vi "Vibration.vi"() -> ()   [LabVIEW 2012]
uses:
  <vilib>/measure/madcrms.llb/Basic Averaged DC-RMS for 1 Chan.vi
  <vilib>/measure/NI_MAPro.lvlib
panel:
  out "选项卡":T1(tab)
  in  "装置IP":string
  in  "?":bool
  in  "灵敏度(mv/g)":u16=1 min=1
  in  "采样率(ksps)":T2(ring)
  in  "?":bool
  in  "?":bool
  in  "开始":bool
  in  "?":bool
  in  "设置装置网关":string
  in  "设置装置子网掩码":string
  in  "设置装置IP":string
  in  "?":bool
  in  "是否开启电流源":u8(knob) scale=0.0..1.0
  in  "是否进行自校准":u8(knob) scale=0.0..1.0
  in  "?":bool
  in  "?":path
  in  "是否保存数据":u8(knob) scale=0.0..1.0
  in  "?":bool
  out "进度条":dbl(slide) scale=0.0..99.0
  out "字符串":string
  out "波形卡":enum32{"波形卡 1", "波形卡 2", "波形卡 3"}(tab)
  in  "AC/DC":bool
  in  "Y轴调整":dbl(knob)=1.0 min=0.0001 max=5.5 step=0.001 scale=0.0001..5.5
  out "?":dbl[](graph)
  out "?":dbl[](graph)
  in  "X轴调整":u16(knob)=50 min=50 max=50000 scale=50.0..50000.0
  in  "列表框":i32(listbox)
  out "?":u16[](graph)
  out "转 \n速":u16(knob) scale=0.0..20000.0
  # "PageUp\nPageDown\n微调"
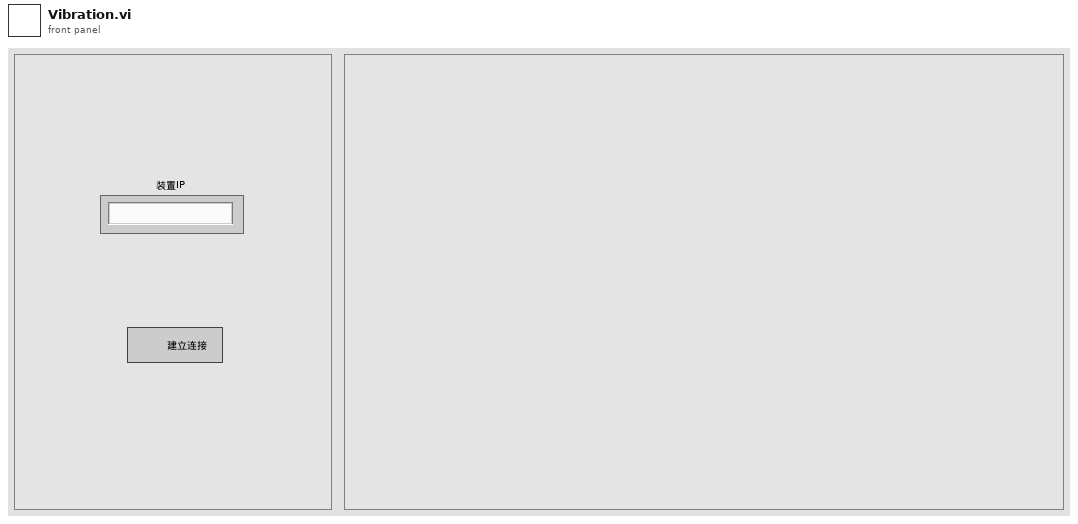
[diagram p1: front panel]
types:
  T1 = enum32{"选项卡 1", "选项卡 2", "选项卡 3", "选项卡 4", "选项卡 5", "选项卡 6", "选项卡 7"}
  T2 = enum16{"105.468", "52.734", "35.156", "26.367", "21.094", "17.578", "15.067", "13.184", "11.719", "10.545"}
  T3 = enum8{"Enabled", "Disabled", "Disabled and Grayed Out"}
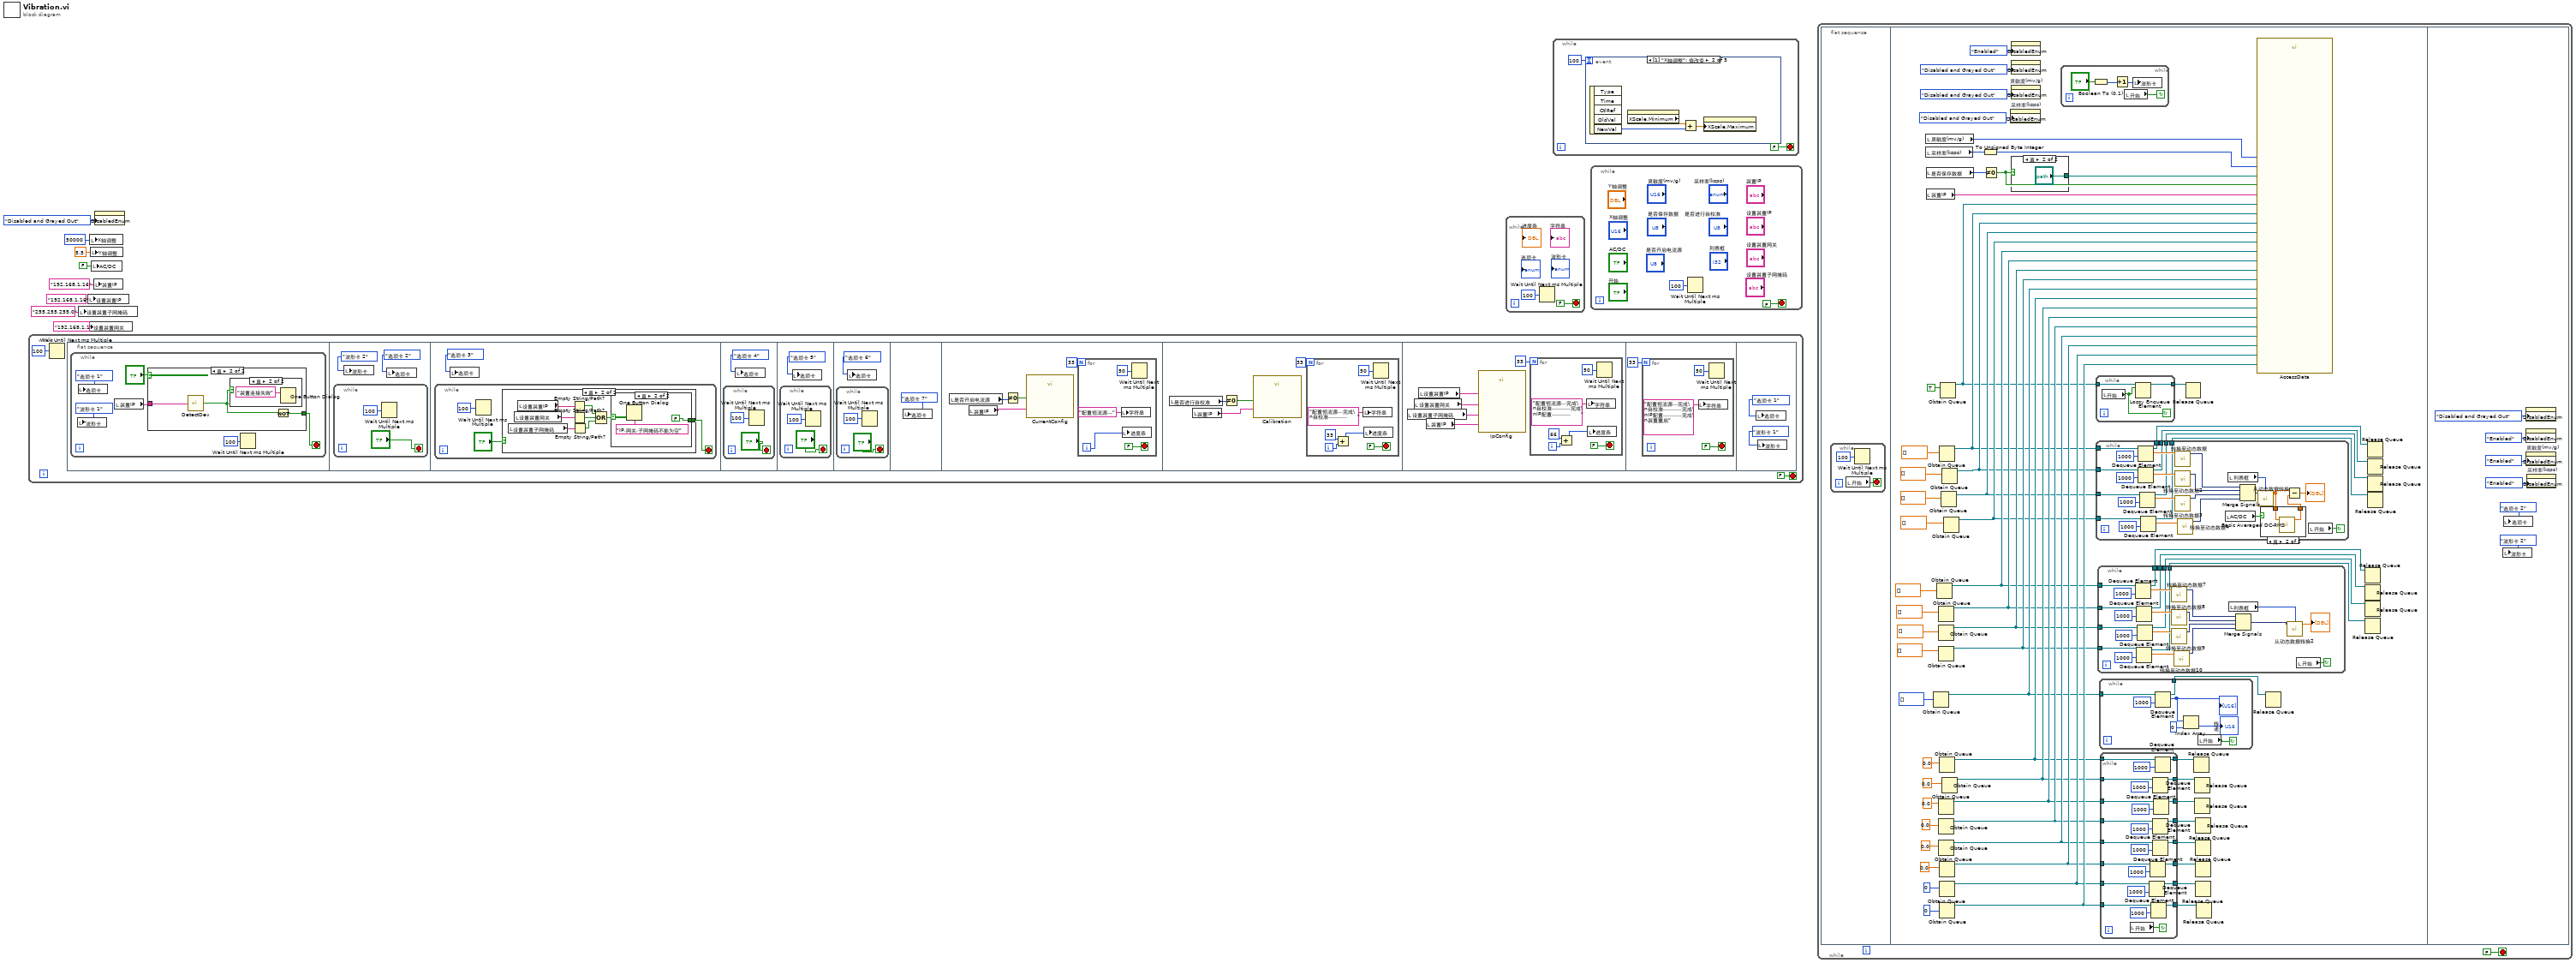
[diagram p0: block diagram]
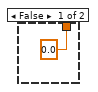
[diagram p2: hidden frame]
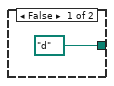
[diagram p3: hidden frame]
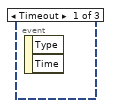
[diagram p4: hidden frame]
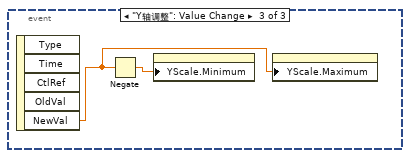
[diagram p5: hidden frame]
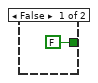
[diagram p6: hidden frame]
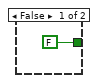
[diagram p8: hidden frame]
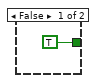
[diagram p9: hidden frame]
diagram:
  n1 = while {
    stop <- FALSE stop-if-true
    n2 = Wait Until Next ms Multiple(millisecond multiple=u32 100 ("毫秒倍数")) -> ()  [unwired: 1 out]
    n3 = flat-sequence {
      frame #0 {
        n4 = while {
          stop <- w15 stop-if-true
          n5 = local write "波形卡"(enum32{"波形卡 1", "波形卡 2", "波形卡 3"}."波形卡 1" ("波形卡")) -> ()
          n6 = local write "选项卡"(T1."选项卡 1" ("选项卡")) -> ()
          n7 = local read "装置IP"() -> (w11:string)
          n8 = case shown="真" "?" {
            tunnel: [FALSE w20] -> w15
            tunnel: w11 -> [_ w18]
            frame False {
            }
            frame True {
              n9 = call "DetectDev.vi"("IP."=w18) -> ("Fail"=w19:bool)
              n10 = case shown="真" w19 {
                frame False {
                }
                frame True {
                  n11 = One Button Dialog(message="装置连接失败" ("消息")) -> ()  [unwired: 1 in, 1 out]
                }
              }
              n12 = Not(x=w19) -> (.not. x?=w20:bool)
            }
          }
          n13 = Wait Until Next ms Multiple(millisecond multiple=u32 100 ("毫秒倍数")) -> ()  [unwired: 1 out]
        }
      }
      frame #1 {
        n14 = while {
          stop <- "?" stop-if-true
          n15 = Wait Until Next ms Multiple(millisecond multiple=u32 100 ("毫秒倍数")) -> ()  [unwired: 1 out]
        }
        n16 = local write "波形卡"(enum32{"波形卡 1", "波形卡 2", "波形卡 3"}."波形卡 2" ("波形卡")) -> ()
        n17 = local write "选项卡"(T1."选项卡 2" ("选项卡")) -> ()
      }
      frame #2 {
        n18 = while {
          stop <- w27 stop-if-true
          n19 = Wait Until Next ms Multiple(millisecond multiple=u32 100 ("毫秒倍数")) -> ()  [unwired: 1 out]
          n20 = case shown="真" "?" {
            tunnel: [FALSE w31] -> w27
            frame False {
            }
            frame True {
              n21 = local read "设置装置子网掩码"() -> (w38:string)
              n22 = local read "设置装置网关"() -> (w37:string)
              n23 = local read "设置装置IP"() -> (w36:string)
              n24 = Empty String/Path?(string/path=w36) -> (empty?=w33:bool)
              n25 = Empty String/Path?(string/path=w37) -> (empty?=w34:bool)
              n26 = Empty String/Path?(string/path=w38) -> (empty?=w35:bool)
              n27 = Compound Arithmetic op=OR(w33, w34, w35) -> (w32:bool)
              n28 = case shown="真" w32 {
                tunnel: [TRUE FALSE] -> w31
                frame False {
                }
                frame True {
                  n29 = One Button Dialog(message="IP,网关,子网掩码不能为空" ("消息")) -> ()  [unwired: 1 in, 1 out]
                }
              }
            }
          }
        }
        n30 = local write "选项卡"(T1."选项卡 3" ("选项卡")) -> ()
      }
      frame #3 {
        n31 = while {
          stop <- "?" stop-if-true
          n32 = Wait Until Next ms Multiple(millisecond multiple=u32 100 ("毫秒倍数")) -> ()  [unwired: 1 out]
        }
        n33 = local write "选项卡"(T1."选项卡 4" ("选项卡")) -> ()
      }
      frame #4 {
        n34 = while {
          stop <- "?" stop-if-true
          n35 = Wait Until Next ms Multiple(millisecond multiple=u32 100 ("毫秒倍数")) -> ()  [unwired: 1 out]
        }
        n36 = local write "选项卡"(T1."选项卡 5" ("选项卡")) -> ()
      }
      frame #5 {
        n37 = while {
          stop <- "?" stop-if-true
          n38 = Wait Until Next ms Multiple(millisecond multiple=u32 100 ("毫秒倍数")) -> ()  [unwired: 1 out]
        }
        n39 = local write "选项卡"(T1."选项卡 6" ("选项卡")) -> ()
      }
      frame #6 {
        n40 = local write "选项卡"(T1."选项卡 7" ("选项卡")) -> ()
      }
      frame #7 {
        n41 = local read "是否开启电流源"() -> (w53:u8)
        n42 = local read "装置IP"() -> (w52:string)
        n43 = Not Equal To 0?(x=w53) -> (x != 0?=w54:bool)
        n44 = call "CurrentConfig.vi"("Current"=w54, "IP"=w52) -> ()
        n45 = for {
          N: 33 -> [_]
          i -> [w56]
          stop <- FALSE stop-if-true
          n46 = local write "字符串"("配置恒流源..." ("字符串")) -> ()
          n47 = local write "进度条"(w56) -> ()
          n48 = Wait Until Next ms Multiple(millisecond multiple=u32 50 ("毫秒倍数")) -> ()  [unwired: 1 out]
        }
      }
      frame #8 {
        n49 = local read "是否进行自校准"() -> (w61:u8)
        n50 = local read "装置IP"() -> (w60:string)
        n51 = Not Equal To 0?(x=w61) -> (x != 0?=w62:bool)
        n52 = call "Calibration.vi"("Enable"=w62, "IP."=w60) -> ()
        n53 = for {
          N: 33 -> [_]
          i -> [w66]
          stop <- FALSE stop-if-true
          n54 = Add(x=33, y=w66) -> (x+y=w65:i32)
          n55 = local write "字符串"("配置恒流源...完成\n自校准...........      " ("字符串")) -> ()
          n56 = local write "进度条"(w65) -> ()
          n57 = Wait Until Next ms Multiple(millisecond multiple=u32 50 ("毫秒倍数")) -> ()  [unwired: 1 out]
        }
      }
      frame #9 {
        n58 = local read "设置装置子网掩码"() -> (w72:string)
        n59 = local read "设置装置网关"() -> (w71:string)
        n60 = local read "设置装置IP"() -> (w70:string)
        n61 = local read "装置IP"() -> (w73:string)
        n62 = call "IpConfig.vi"("Gateway"=w71, "SubnetMask"=w72, "IP"=w70, "CurrentIP"=w73) -> ()
        n63 = for {
          N: 33 -> [_]
          i -> [w77]
          stop <- FALSE stop-if-true
          n64 = Add(x=66, y=w77) -> (x+y=w76:i32)
          n65 = local write "字符串"("配置恒流源...完成\n自校准...........完成\nIP配置...........      " ("字符串")) -> ()
          n66 = local write "进度条"(w76) -> ()
          n67 = Wait Until Next ms Multiple(millisecond multiple=u32 50 ("毫秒倍数")) -> ()  [unwired: 1 out]
        }
      }
      frame #10 {
        n68 = for {
          N: 33 -> [_]
          stop <- FALSE stop-if-true
          n69 = local write "字符串"("配置恒流源...完成\n自校准...........完成\nIP配置...........完成\n装置重启" ("字符串")) -> ()
          n70 = Wait Until Next ms Multiple(millisecond multiple=u32 50 ("毫秒倍数")) -> ()  [unwired: 1 out]
        }
      }
      frame #11 {
        n71 = local write "选项卡"(T1."选项卡 1" ("选项卡")) -> ()
        n72 = local write "波形卡"(enum32{"波形卡 1", "波形卡 2", "波形卡 3"}."波形卡 1" ("波形卡")) -> ()
      }
    }
  }
  n73 = local write "设置装置子网掩码"("255.255.255.0" ("新子网掩码")) -> ()
  n74 = local write "设置装置网关"("192.168.1.1" ("新网关")) -> ()
  n75 = local write "设置装置IP"("192.168.1.16" ("新装置IP")) -> ()
  n76 = local write "X轴调整"(u16 50000 ("X轴调整")) -> ()
  n77 = local write "Y轴调整"(5.5 ("Y轴调整")) -> ()
  n78 = local write "AC/DC"(FALSE ("AC/DC")) -> ()
  n79 = local write "装置IP"("192.168.1.16" ("装置IP")) -> ()
  n80 = property class="Bool (严格)"("DisabledEnum"=T3."Disabled and Grayed Out" ("禁用")) -> ()  [unwired: 2 in, 2 out]
  n81 = while {
    stop <- FALSE stop-if-true
    n82 = Wait Until Next ms Multiple(millisecond multiple=u32 100 ("毫秒倍数")) -> ()  [unwired: 1 out]
  }
  n83 = while {
    stop <- FALSE stop-if-true
    n84 = event shown="[1] \"X轴调整\": 值改变" {
      selector: _ -> [_ _ _]
      dyn-events: _ -> [_ _ _]
      timeout: 100 -> [_ _ _]
      event Timeout {
        n85 = event-data() -> ()  [unwired: 1 in, 2 out]
      }
      event "X轴调整": Value Change {
        n86 = event-data() -> ("NewVal"=w93:u16)  [unwired: 1 in, 4 out]
        n87 = property class="WFChart (严格)"() -> ("XScale.Minimum"=w92:dbl)  [unwired: 2 in, 2 out]
        n88 = Add(x=w92, y=w93) -> (x+y=w91:dbl)
        n89 = property class="WFChart (严格)"("XScale.Maximum"=w91) -> ()  [unwired: 2 in, 2 out]
      }
      event "Y轴调整": Value Change {
        n90 = event-data() -> ("NewVal"=w94:dbl)  [unwired: 1 in, 4 out]
        n91 = Negate(x=w94) -> (-x=w95:dbl)
        n92 = property class="WFChart (严格)"("YScale.Minimum"=w95) -> ()  [unwired: 2 in, 2 out]
        n93 = property class="WFChart (严格)"("YScale.Maximum"=w94) -> ()  [unwired: 2 in, 2 out]
      }
    }
  }
  n94 = while {
    stop <- FALSE stop-if-true
    n95 = Wait Until Next ms Multiple(millisecond multiple=u32 100 ("毫秒倍数")) -> ()  [unwired: 1 out]
  }
  n96 = while {
    stop <- FALSE stop-if-true
    n97 = flat-sequence {
      frame #0 {
        n98 = while {
          stop <- w99 stop-if-true
          n99 = local read "开始"() -> (w99:bool)
          n100 = Wait Until Next ms Multiple(millisecond multiple=u32 100 ("毫秒倍数")) -> ()  [unwired: 1 out]
        }
      }
      frame #1 {
        n101 = local read "灵敏度(mv/g)"() -> (w146:u16)
        n102 = local read "采样率(ksps)"() -> (w145:T2)
        n103 = local read "是否保存数据"() -> (w144:u8)
        n104 = local read "装置IP"() -> (w142:string)
        n105 = Obtain Queue(element data type=u16[] [] ("无符号16位整型")) -> (queue out=w110:refnum<queue>)  [unwired: 4 in, 2 out]
        n106 = Obtain Queue(element data type=dbl[] [] ("Amp Spectrum Mag (Vrms)")) -> (queue out=w106:refnum<queue>)  [unwired: 4 in, 2 out]
        n107 = Obtain Queue(element data type=0.0) -> (queue out=w113:refnum<queue>)  [unwired: 4 in, 2 out]
        n108 = Obtain Queue(element data type=dbl[] [] ("Amp Spectrum Mag (Vrms)")) -> (queue out=w107:refnum<queue>)  [unwired: 4 in, 2 out]
        n109 = Obtain Queue(element data type=dbl[] [] ("Amp Spectrum Mag (Vrms)")) -> (queue out=w108:refnum<queue>)  [unwired: 4 in, 2 out]
        n110 = Obtain Queue(element data type=dbl[] [] ("Amp Spectrum Mag (Vrms)")) -> (queue out=w109:refnum<queue>)  [unwired: 4 in, 2 out]
        n111 = Obtain Queue(element data type=0.0) -> (queue out=w114:refnum<queue>)  [unwired: 4 in, 2 out]
        n112 = Obtain Queue(element data type=0.0) -> (queue out=w115:refnum<queue>)  [unwired: 4 in, 2 out]
        n113 = Obtain Queue(element data type=dbl[] [] ("16位整型")) -> (queue out=w102:refnum<queue>)  [unwired: 4 in, 2 out]
        n114 = Obtain Queue(element data type=u8 0) -> (queue out=w117:refnum<queue>)  [unwired: 4 in, 2 out]
        n115 = Obtain Queue(element data type=0.0) -> (queue out=w111:refnum<queue>)  [unwired: 4 in, 2 out]
        n116 = Obtain Queue(element data type=0.0) -> (queue out=w116:refnum<queue>)  [unwired: 4 in, 2 out]
        n117 = Obtain Queue(element data type=u8 0) -> (queue out=w118:refnum<queue>)  [unwired: 4 in, 2 out]
        n118 = Obtain Queue(element data type=TRUE) -> (queue out=w101:refnum<queue>)  [unwired: 4 in, 2 out]
        n119 = Obtain Queue(element data type=dbl[] [] ("16位整型")) -> (queue out=w104:refnum<queue>)  [unwired: 4 in, 2 out]
        n120 = Obtain Queue(element data type=dbl[] [] ("16位整型")) -> (queue out=w103:refnum<queue>)  [unwired: 4 in, 2 out]
        n121 = Obtain Queue(element data type=0.0) -> (queue out=w112:refnum<queue>)  [unwired: 4 in, 2 out]
        n122 = Obtain Queue(element data type=dbl[] [] ("16位整型")) -> (queue out=w105:refnum<queue>)  [unwired: 4 in, 2 out]
        n123 = To Unsigned Byte Integer(number=w145) -> (unsigned 8bit integer=w149:u8)
        n124 = Not Equal To 0?(x=w144) -> (x != 0?=w147:bool)
        n125 = property on="采样率(ksps)" class="Enum (严格)"("DisabledEnum"=T3."Disabled and Grayed Out" ("禁用")) -> ()  [unwired: 2 in, 2 out]
        n126 = property class="Bool (严格)"("DisabledEnum"=T3."Enabled" ("禁用")) -> ()  [unwired: 2 in, 2 out]
        n127 = property class="Bool"("DisabledEnum"=T3."Disabled and Grayed Out" ("禁用")) -> ()  [unwired: 2 in, 2 out]
        n128 = property on="灵敏度(mv/g)" class="DigNum (严格)"("DisabledEnum"=T3."Disabled and Grayed Out" ("禁用")) -> ()  [unwired: 2 in, 2 out]
        n129 = case shown="真" w147 {
          tunnel: [path "d:/" ("路径（使用对话框）") "?"] -> w148
          frame False {
          }
          frame True {
          }
        }
        n130 = while {
          stop <- w169 continue-if-true
          n131 = Boolean To (0,1)(Boolean="?") -> (0, 1=w172:i16)
          n132 = Increment(x=w172) -> (x+1=w170:i16)
          n133 = local read "开始"() -> (w169:bool)
          n134 = local write "波形卡"(w170) -> ()
        }
        n135 = while {
          tunnel: w101 -> [w168]
          tunnel: [w166] -> w136
          stop <- w167 continue-if-true
          n136 = local read "开始"() -> (w167:bool)
          n137 = Lossy Enqueue Element(queue=w168, element=w167) -> (queue out=w166:refnum<queue>)  [unwired: 1 in, 3 out]
        }
        n138 = while {
          tunnel: w102 -> [w206]
          tunnel: w103 -> [w205]
          tunnel: w104 -> [w204]
          tunnel: w105 -> [w203]
          tunnel: [w183] -> w120
          tunnel: [w182] -> w121
          tunnel: [w181] -> w122
          tunnel: [w180] -> w123
          stop <- w188 continue-if-true
          n139 = Dequeue Element(queue=w206, timeout in ms (-1)=1000 ("超时毫秒(-1)")) -> (queue out=w183:refnum<queue>, element=w196:dbl[])  [unwired: 1 in, 2 out]
          n140 = Dequeue Element(queue=w205, timeout in ms (-1)=1000 ("超时毫秒(-1)")) -> (queue out=w182:refnum<queue>, element=w202:dbl[])  [unwired: 1 in, 2 out]
          n141 = Dequeue Element(queue=w204, timeout in ms (-1)=1000 ("超时毫秒(-1)")) -> (queue out=w181:refnum<queue>, element=w200:dbl[])  [unwired: 1 in, 2 out]
          n142 = Dequeue Element(queue=w203, timeout in ms (-1)=1000 ("超时毫秒(-1)")) -> (queue out=w180:refnum<queue>, element=w198:dbl[])  [unwired: 1 in, 2 out]
          n143 = call "转换至动态数据"("Array"=w196) -> ("Dynamic Data Type"=w195:dynamicdata)  [unwired: 3 in]
          n144 = call "转换至动态数据2"("Array"=w202) -> ("Dynamic Data Type"=w201:dynamicdata)  [unwired: 3 in]
          n145 = call "转换至动态数据3"("Array"=w200) -> ("Dynamic Data Type"=w199:dynamicdata)  [unwired: 3 in]
          n146 = call "转换至动态数据4"("Array"=w198) -> ("Dynamic Data Type"=w197:dynamicdata)  [unwired: 3 in]
          n147 = local read "AC/DC"() -> (w189:bool)
          n148 = local read "列表框"() -> (w194:i32)
          n149 = Merge Signals(w195, w201, w199, w197) -> (w193:dynamicdata)
          n150 = call "从动态数据转换"("Dynamic Data Type"=w193, "Channel"=w194) -> ("Array"=w192:dbl[])  [unwired: 2 in]
          n151 = case shown="真" w189 {
            tunnel: w192 -> [_ w209]
            tunnel: [0.0 ("DC value") w208] -> w191
            frame False {
            }
            frame True {
              n152 = call-poly <vilib>:"Basic Averaged DC-RMS.vi"("signal in"=w209) -> ("DC value"=w208:dbl)  [unwired: 7 in, 3 out]
            }
          }
          n153 = Subtract(x=w192, y=w191) -> (x-y=→"?":dbl[])
          n154 = local read "开始"() -> (w188:bool)
        }
        n155 = while {
          tunnel: w106 -> [w258]
          tunnel: w107 -> [w257]
          tunnel: w108 -> [w256]
          tunnel: w109 -> [w255]
          tunnel: [w238] -> w124
          tunnel: [w237] -> w125
          tunnel: [w236] -> w126
          tunnel: [w235] -> w127
          stop <- w243 continue-if-true
          n156 = Dequeue Element(queue=w258, timeout in ms (-1)=1000 ("超时毫秒(-1)")) -> (queue out=w238:refnum<queue>, element=w254:dbl[])  [unwired: 1 in, 2 out]
          n157 = Dequeue Element(queue=w257, timeout in ms (-1)=1000 ("超时毫秒(-1)")) -> (queue out=w237:refnum<queue>, element=w252:dbl[])  [unwired: 1 in, 2 out]
          n158 = Dequeue Element(queue=w255, timeout in ms (-1)=1000 ("超时毫秒(-1)")) -> (queue out=w235:refnum<queue>, element=w248:dbl[])  [unwired: 1 in, 2 out]
          n159 = Dequeue Element(queue=w256, timeout in ms (-1)=1000 ("超时毫秒(-1)")) -> (queue out=w236:refnum<queue>, element=w250:dbl[])  [unwired: 1 in, 2 out]
          n160 = call "转换至动态数据8"("Array"=w252) -> ("Dynamic Data Type"=w251:dynamicdata)  [unwired: 3 in]
          n161 = call "转换至动态数据9"("Array"=w250) -> ("Dynamic Data Type"=w249:dynamicdata)  [unwired: 3 in]
          n162 = call "转换至动态数据7"("Array"=w254) -> ("Dynamic Data Type"=w253:dynamicdata)  [unwired: 3 in]
          n163 = call "转换至动态数据10"("Array"=w248) -> ("Dynamic Data Type"=w247:dynamicdata)  [unwired: 3 in]
          n164 = local read "列表框"() -> (w245:i32)
          n165 = Merge Signals(w253, w251, w249, w247) -> (w244:dynamicdata)
          n166 = call "从动态数据转换2"("Dynamic Data Type"=w244, "Channel"=w245) -> ("Array"=→"?":dbl[])  [unwired: 2 in]
          n167 = local read "开始"() -> (w243:bool)
        }
        n168 = while {
          tunnel: w110 -> [w176]
          tunnel: [w173] -> w119
          stop <- w175 continue-if-true
          n169 = Dequeue Element(queue=w176, timeout in ms (-1)=1000 ("超时毫秒(-1)")) -> (queue out=w173:refnum<queue>, element=w179:u16[])  [unwired: 1 in, 2 out]
          "?" <- w179
          n170 = Index Array(array=w179, index=0 ("索引")) -> (element=→"转 \n速":u16)
          n171 = local read "开始"() -> (w175:bool)
        }
        n172 = while {
          tunnel: w111 -> [w234]
          tunnel: w112 -> [w233]
          tunnel: w113 -> [w232]
          tunnel: w114 -> [w231]
          tunnel: w115 -> [w230]
          tunnel: w116 -> [w229]
          tunnel: w117 -> [w228]
          tunnel: w118 -> [w227]
          tunnel: [w217] -> w135
          tunnel: [w216] -> w134
          tunnel: [w215] -> w133
          tunnel: [w214] -> w132
          tunnel: [w213] -> w131
          tunnel: [w212] -> w130
          tunnel: [w211] -> w129
          tunnel: [w210] -> w128
          stop <- w226 continue-if-true
          n173 = local read "开始"() -> (w226:bool)
          n174 = Dequeue Element(queue=w228, timeout in ms (-1)=1000 ("超时毫秒(-1)")) -> (queue out=w216:refnum<queue>)  [unwired: 1 in, 3 out]
          n175 = Dequeue Element(queue=w229, timeout in ms (-1)=1000 ("超时毫秒(-1)")) -> (queue out=w215:refnum<queue>)  [unwired: 1 in, 3 out]
          n176 = Dequeue Element(queue=w227, timeout in ms (-1)=1000 ("超时毫秒(-1)")) -> (queue out=w217:refnum<queue>)  [unwired: 1 in, 3 out]
          n177 = Dequeue Element(queue=w233, timeout in ms (-1)=1000 ("超时毫秒(-1)")) -> (queue out=w211:refnum<queue>)  [unwired: 1 in, 3 out]
          n178 = Dequeue Element(queue=w231, timeout in ms (-1)=1000 ("超时毫秒(-1)")) -> (queue out=w213:refnum<queue>)  [unwired: 1 in, 3 out]
          n179 = Dequeue Element(queue=w230, timeout in ms (-1)=1000 ("超时毫秒(-1)")) -> (queue out=w214:refnum<queue>)  [unwired: 1 in, 3 out]
          n180 = Dequeue Element(queue=w232, timeout in ms (-1)=1000 ("超时毫秒(-1)")) -> (queue out=w212:refnum<queue>)  [unwired: 1 in, 3 out]
          n181 = Dequeue Element(queue=w234, timeout in ms (-1)=1000 ("超时毫秒(-1)")) -> (queue out=w210:refnum<queue>)  [unwired: 1 in, 3 out]
        }
        n182 = Release Queue(queue=w136) -> ()  [unwired: 2 in, 3 out]
        n183 = Release Queue(queue=w128) -> ()  [unwired: 2 in, 3 out]
        n184 = Release Queue(queue=w129) -> ()  [unwired: 2 in, 3 out]
        n185 = Release Queue(queue=w130) -> ()  [unwired: 2 in, 3 out]
        n186 = Release Queue(queue=w131) -> ()  [unwired: 2 in, 3 out]
        n187 = Release Queue(queue=w132) -> ()  [unwired: 2 in, 3 out]
        n188 = Release Queue(queue=w133) -> ()  [unwired: 2 in, 3 out]
        n189 = Release Queue(queue=w134) -> ()  [unwired: 2 in, 3 out]
        n190 = Release Queue(queue=w135) -> ()  [unwired: 2 in, 3 out]
        n191 = call "AccessData.vi"("Vibration_Channel4_FFT"=w109, "Vibration_Channel3_FFT"=w108, "Vibration_Channel2_FFT"=w107, "Vibration_Channel1_FFT"=w106, "Vibration_Channel1"=w102, "Vibration_Channel2"=w103, "Vibration_Channel3"=w104, "Vibration_Channel4"=w105, "created path"=w148, "Speed_Channel"=w110, "IP地址"=w142, "PRE_Scaler"=w149, "SAVE?"=w147, "Sensitivity"=w146, "Run"=w101, "Temperature_Channel1"=w111, "Temperature_Channel2"=w112, "Temperature_Channel3"=w113, "Temperature_Channel4"=w114, "Temperature_Channel5"=w115, "Temperature_Channel6"=w116, "Temperature_Channel7"=w117, "Humidity_Channel"=w118) -> ()  [unwired: 5 in]
        n192 = Release Queue(queue=w119) -> ()  [unwired: 2 in, 3 out]
        n193 = Release Queue(queue=w124) -> ()  [unwired: 2 in, 3 out]
        n194 = Release Queue(queue=w125) -> ()  [unwired: 2 in, 3 out]
        n195 = Release Queue(queue=w126) -> ()  [unwired: 2 in, 3 out]
        n196 = Release Queue(queue=w127) -> ()  [unwired: 2 in, 3 out]
        n197 = Release Queue(queue=w120) -> ()  [unwired: 2 in, 3 out]
        n198 = Release Queue(queue=w121) -> ()  [unwired: 2 in, 3 out]
        n199 = Release Queue(queue=w122) -> ()  [unwired: 2 in, 3 out]
        n200 = Release Queue(queue=w123) -> ()  [unwired: 2 in, 3 out]
      }
      frame #2 {
        n201 = local write "波形卡"(enum32{"波形卡 1", "波形卡 2", "波形卡 3"}."波形卡 2" ("波形卡")) -> ()
        n202 = local write "选项卡"(T1."选项卡 2" ("选项卡")) -> ()
        n203 = property class="Bool (严格)"("DisabledEnum"=T3."Disabled and Grayed Out" ("禁用")) -> ()  [unwired: 2 in, 2 out]
        n204 = property class="Bool"("DisabledEnum"=T3."Enabled" ("禁用")) -> ()  [unwired: 2 in, 2 out]
        n205 = property on="灵敏度(mv/g)" class="DigNum (严格)"("DisabledEnum"=T3."Enabled" ("禁用")) -> ()  [unwired: 2 in, 2 out]
        n206 = property on="采样率(ksps)" class="Enum (严格)"("DisabledEnum"=T3."Enabled" ("禁用")) -> ()  [unwired: 2 in, 2 out]
      }
    }
  }
